vi "SortPhases.vi"(8 "error in (no error)":errorcluster, 10 "PmuReport":T1 {"Synx" format="%#_4g"; "Timestamp" format="%.6f"}, 11 "C37.118 PMU in":refnum<class "C37.118 PMU.lvclass">) -> (0 "error out":errorcluster, 2 "PmuReport 2":T1 {"Synx" format="%#_4g"; "Timestamp" format="%.6f"}, 3 "C37.118 PMU out":refnum<class "C37.118 PMU.lvclass">)   [LabVIEW 2018, in "SensorPlugins.lvlib" / "C37.118 PMU.lvclass"]
uses:
  C37.118 PMU.lvclass
  C:/projects/ICDAS/NistPluggableModules/Sensor/SensorPlugins/PmuBaseClass/PmuBase.lvclass
  PmuBaseClass/Typedef/PmuData.ctl
  PmuBaseClass/PmuBase.lvclass/PmuBase.ctl
  PmuBaseClass/Typedef/ePhases.ctl
  PmuBaseClass/Accessors/Read PhaseArray.vi
  PmuBaseClass/PmuBase.lvclass
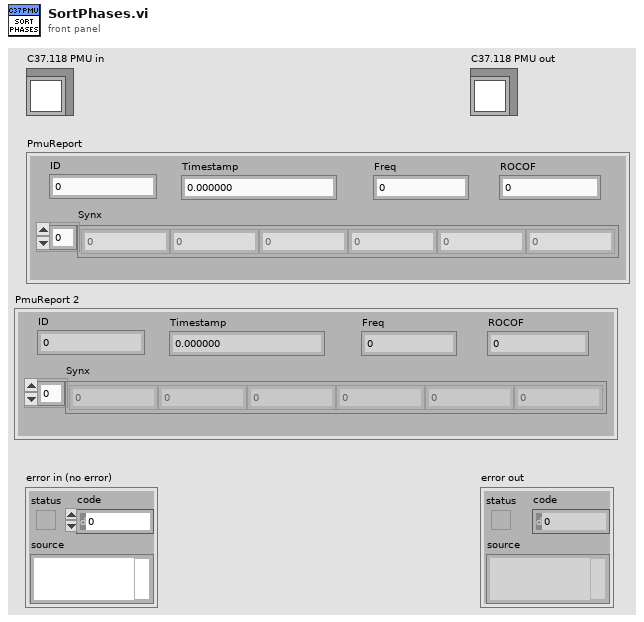
[diagram p1: front panel]
types:
  T1 = typedef "SensorPlugins.lvlib/PmuBase.lvclass/PmuData.ctl" = cluster{"Timestamp":dbl, "Synx":cdb[], "Freq":dbl, "ROCOF":dbl, "ID":i16}
  T2 = typedef "SensorPlugins.lvlib/PmuBase.lvclass/ePhases.ctl" = enum16{"VA", "VB", "VC", "V+", "IA", "IB", "IC", "I+", "none"}
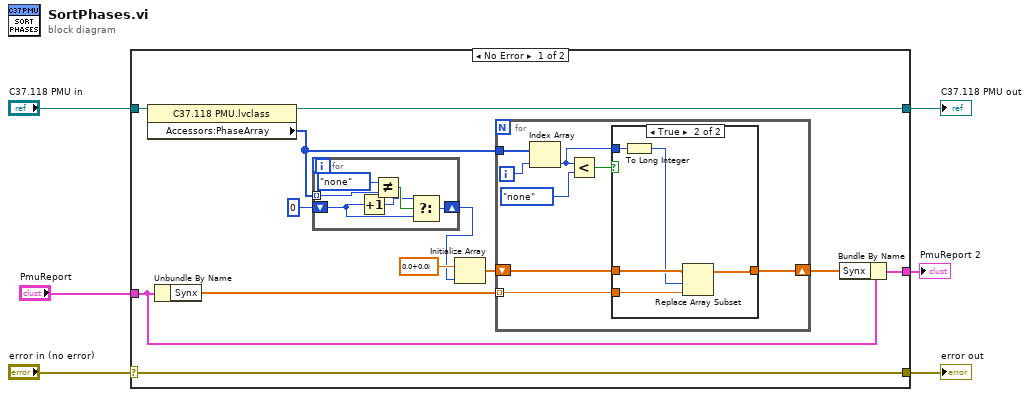
[diagram p0: block diagram]
diagram:
  n1 = case shown="No Error" "error in (no error)" {
    selector: "error in (no error)" -> [w17 w41]
    tunnel: [w17 w41] -> w5
    tunnel: [w16 w40] -> w3
    tunnel: "C37.118 PMU in" -> [w18 w40]
    tunnel: "PmuReport" -> [w9 w39]
    tunnel: [w7 w39] -> w1
    frame No Error {
      n2 = property class="C37.118 PMU.lvclass"(reference=w18) -> (reference out=w16:refnum<class "C37.118 PMU.lvclass">, "Accessors:PhaseArray"=w12:T2[])  [unwired: 1 in, 1 out]
      n3 = Unbundle By Name(w9) -> ("Synx"=w14:cdb[])
      n4 = for {
        tunnel: w12 -> [w24] mode=indexing
        shift-right: [w19] -> w10
        shift-left: 0 -> [w21]
        n5 = Increment(x=w21) -> (x+1=w20:i32)
        n6 = Not Equal?(x=ePhases."none", y=w24) -> (x != y?=w22:bool)
        n7 = Select(t=w20, s=w22, f=w21) -> (s? t:f=w19:i32)
      }
      n8 = Initialize Array(cdb 0.0+0.0i ("element"), w10) -> (w13:cdb[])
      n9 = for {
        tunnel: w12 -> [w32]
        tunnel: w14 -> [w25] mode=indexing
        shift-right: [w26] -> w8
        shift-left: w13 -> [w27]
        i -> [w31]
        n10 = Index Array(array=w32, index=w31) -> (element=w28:T2)
        n11 = Less?(x=w28, y=ePhases."none") -> (x < y?=w29:bool)
        n12 = case shown="True" w29 {
          tunnel: w28 -> [_ w38]
          tunnel: w27 -> [w33 w37]
          tunnel: [w33 w35] -> w26
          tunnel: w25 -> [_ w36]
          frame False {
          }
          frame True {
            n13 = To Long Integer(number=w38) -> (32bit integer=w34:i32)
            n14 = Replace Array Subset(array=w37, new element=w36, index=w34) -> (w35:cdb[])
          }
        }
      }
      n15 = Bundle By Name(cluster=w9, "Synx"=w8) -> (w7:T1)
    }
    frame Error {
    }
  }
  "error out" <- w5
  "C37.118 PMU out" <- w3
  "PmuReport 2" <- w1
